vi "BRig_dataCurrent_targetBUR.vi"() -> (2 "output_targetBUR":i32)   [LabVIEW 2014]
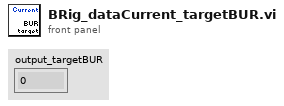
[diagram p1: front panel]
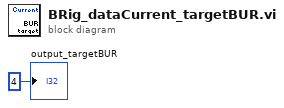
[diagram p0: block diagram]
diagram:
  "output_targetBUR" <- 4 ("output_iBlock")
